vi "Missing System Array 1.vi"() -> ()   [LabVIEW 2009]
panel:
  out "System Array":void[](array[numeric])
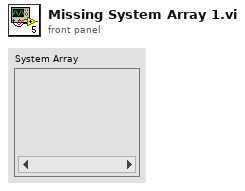
[diagram p1: front panel]
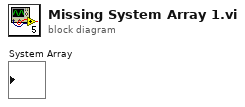
[diagram p0: block diagram]
diagram:
